vi "Filter.vi"(6 "Show Hierarhy":T1={"Show hierarhy in first column(F)"=FALSE, "Left separator"="[", "Right separator"="] "}, 8 "Error out":errorcluster, 9 "Column":i32, 10 "Filter":string, 11 "Tree in":refnum<class "Tree.lvclass">) -> (0 "Error out":errorcluster, 3 "Tree out":refnum<class "Tree.lvclass">)   [LabVIEW 2021, in "Tree.lvlib" / "Tree.lvclass"]
uses:
  Tree.lvclass
  Private/TreeControllerTag.ctl
  Tree.lvclass/Tree.ctl
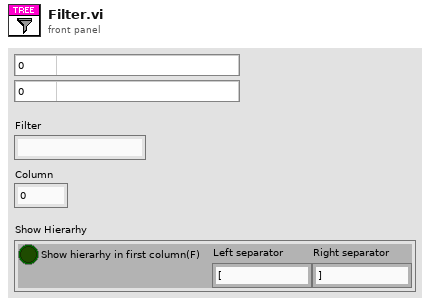
[diagram p1: front panel]
types:
  T1 = cluster{"Show hierarhy in first column(F)":bool, "Left separator":string, "Right separator":string}
  T2 = typedef "Tree.lvlib/Tree.lvclass/TreeControllerTag.ctl" = enum8{"Null", "1. Add item", "2. Delete item", "3. Get All Tree Data", "4. Drag Starting", "5. Drag Ended", "6. Add Tree Values", "7. Get Item Value", "8. Edit Item", "9. StepBack", "10. Filter"}
  T3 = cluster{"Filter":string, "Column":i32, "Show Hierarhy":cluster{"Show hierarhy in first column(F)":bool, "Left separator":string, "Right separator":string}}
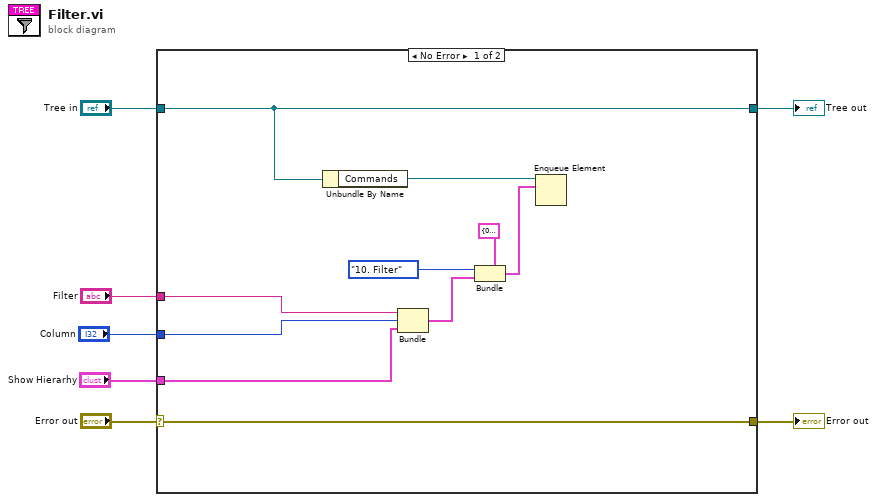
[diagram p0: block diagram]
diagram:
  n1 = case shown="No Error" "Error out" {
    selector: "Error out" -> [w17 w19]
    tunnel: [w17 w19] -> w6
    tunnel: [w15 w18] -> w4
    tunnel: "Tree in" -> [w15 w18]
    tunnel: "Filter" -> [w11 _]
    tunnel: "Column" -> [w10 _]
    tunnel: "Show Hierarhy" -> [w8 _]
    frame No Error {
      n2 = Unbundle By Name(w15) -> ("Commands"=w16:refnum<queue>)
      n3 = Bundle("Filter"=w11, "Column"=w10, "Show Hierarhy"=w8) -> (w9:T3)  [unwired: 1 in]
      n4 = Bundle(cluster=cluster{"Tag":u8, "Value":variant} {"Tag"=0, "Value"=variant} ("element"), "Tag"=TreeControllerTag."10. Filter", "Value"=w9) -> (w13:cluster{"Tag":u8, "Value":variant})
      n5 = Enqueue Element(queue=w16, element=w13) -> ()  [unwired: 2 in, 3 out]
    }
    frame Error {
    }
  }
  "Error out" <- w6
  "Tree out" <- w4
